vi "Create Test from Pointer.vi"() -> (3 "Test":refnum<class "Executioner.lvclass">)   [LabVIEW 2019, in "Mock Executioner.lvclass"]
uses:
  <vilib>/gpm_packages/@cs/test-executive/Source/Sandbox/While Loop Stop Example/Mock Executioner/Mock Executioner.lvclass
  <vilib>/gpm_packages/@cs/test-executive/Source/Test Executive/Executioner/Executioner.lvclass
  C:/Program Files/National Instruments/LabVIEW 2019/vi.lib/gpm_packages/@cs/test-executive/Source/Test Executive/Executioner/Executioner.lvclass
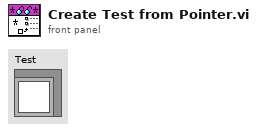
[diagram p1: front panel]
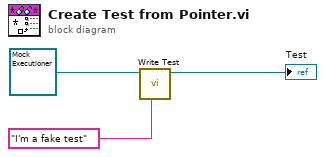
[diagram p0: block diagram]
diagram:
  n1 = call <vilib>:"Write Test.vi"("Test"="I'm a fake test", "Executioner in"=refnum<class "Mock Executioner.lvclass"> refnum ("Mock Executioner.lvclass")) -> ("Executioner out"=→"Test":refnum<class "Mock Executioner.lvclass">)  [unwired: 9 in]
